vi "ClientGUIGraph.vi"() -> ()   [LabVIEW 2021]
doc: "Le protocole UDP diffère du protocole TCP car il n'y a pas de détection d'erreur avec les paquets d'informations qui sont envoyés ; il n'y a donc aucune garantie qu'un destinataire reçoive bien des données.\n\nLe protocole UDP offre la possibilité de diffuser des données sur un réseau. Spécifiez simplement une adresse IP de uns (255.255.255.255) pour essayer de diffuser l'information sur tout le réseau. Gardez à l'esprit que des routeurs et d'autres périphériques de réseau refusent généralement de diffuser au-delà de certains points, la diffusion est donc limitée dans la pratique."
panel:
  in  "Période\n(en ms)":u32(slide)=100 min=5 max=100 step=5 scale=5.0..100.0
  in  "Instruction\n[1] Get Analog\n[2] Set Digital (PWM)":u8=1 min=1 max=2
  in  "Value [0 - 255]":u8=1
  in  "Pin [0 - 11]":u8=1 max=11
  out "Request Command":u8[](array[numeric])
  out "Value":u16
  out "?":u16(graph)
  out "Response Command":u8[](array[numeric])
  in  "?":bool
  # "Version"
  # "Version"
  # "Instruction"
  # "Argument[0]"
  # "Argument[1]"
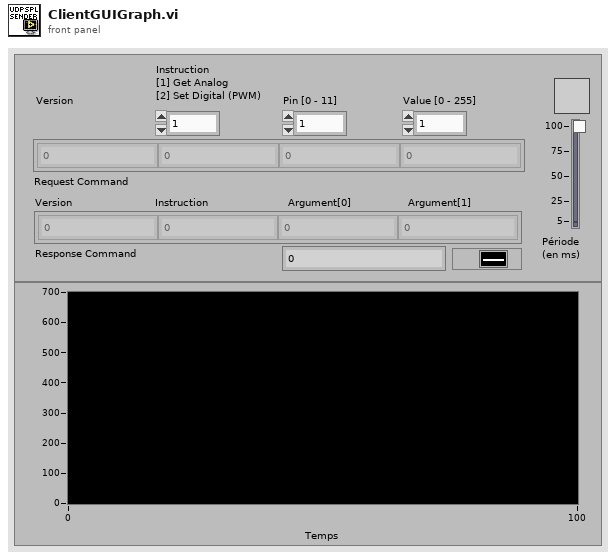
[diagram p1: front panel]
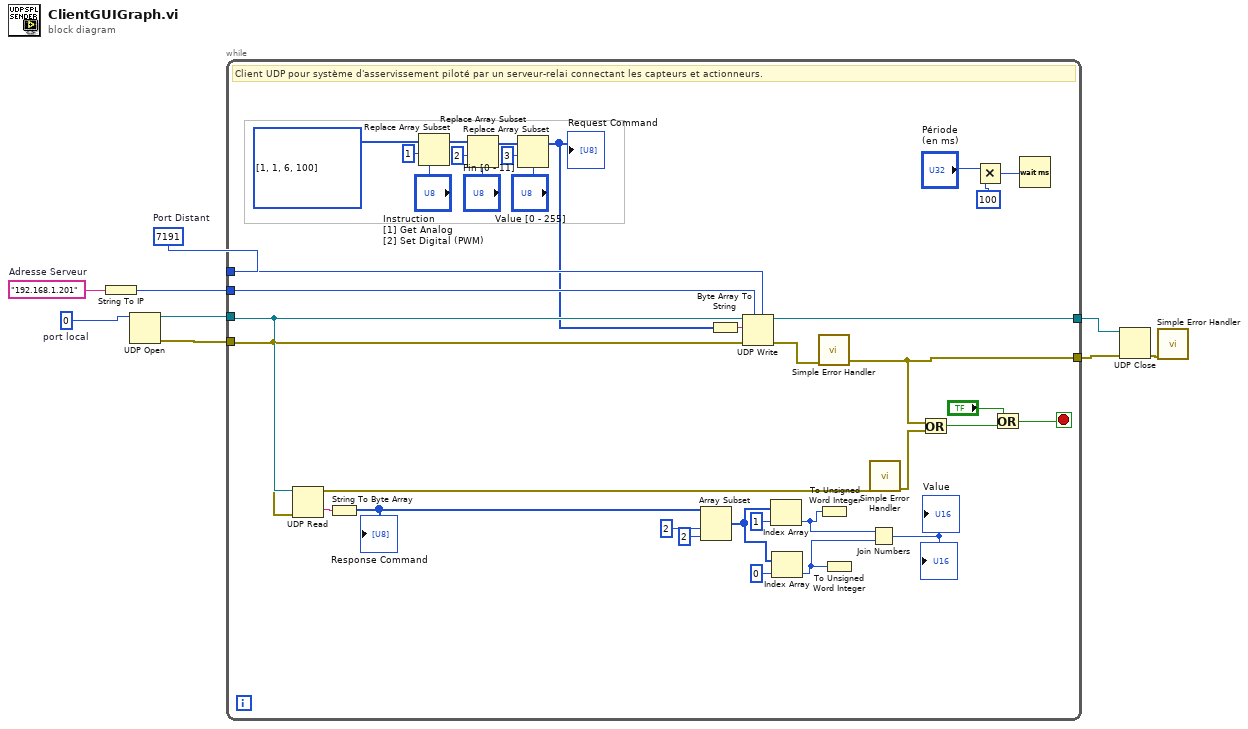
[diagram p0: block diagram]
diagram:
  w2 = u16 7191  # Port Distant
  w6 = u16 0  # port local
  w9 = "192.168.1.201"  # Adresse Serveur
  n1 = String To IP(1:w9) -> (0:w1:u32)
  n2 = UDP Open(11:w6) -> (port=w8:refnum<k16>, 0:w7:errorcluster)  [unwired: 4 in, 1 out]
  n3 = while {
    tunnel: w8 -> [w43]
    tunnel: w7 -> [w34]
    tunnel: w2 -> [w45]
    tunnel: [w29] -> w5
    tunnel: [w28] -> w4
    tunnel: w1 -> [w26]
    stop <- w27 stop-if-true
    # "Client UDP pour système d'asservissement piloté par un serveur-relai connectant les capteurs et actionneurs."
    n4 = UDP Read(connection ID=w43, 8:w34) -> (data out=w42:string, error out=w25:errorcluster)  [unwired: 2 in, 3 out]
    n5 = String To Byte Array(string=w42) -> (unsigned byte array=w10:u8[])
    "Response Command" <- w10
    n6 = Replace Array Subset(array=u8[] [1, 1, 6, 100], new element="Instruction\n[1] Get Analog\n[2] Set Digital (PWM)", index=1 ("indice")) -> (w20:u8[])
    n7 = Replace Array Subset(array=w20, new element="Pin [0 - 11]", index=2 ("indice")) -> (w19:u8[])
    n8 = Replace Array Subset(array=w19, new element="Value [0 - 255]", index=3 ("indice")) -> (w15:u8[])
    "Request Command" <- w15
    n9 = Array Subset(array=w10, index=2 ("indice"), length=2 ("longueur")) -> (w37:u8[])
    n10 = Byte Array To String(unsigned byte array=w15) -> (string=w44:string)
    n11 = UDP Write(address=w26, port or service name=w45, connection ID=w43, data in=w44, 8:w34) -> (error out=w31:errorcluster, 3:w28:refnum<k16>)  [unwired: 1 in]
    n12 = Index Array(array=w37, index=1 ("indice")) -> (element=w36:u8)
    n13 = Index Array(array=w37, index=0 ("indice")) -> (element=w35:u8)
    n14 = call <vilib>:"Simple Error Handler.vi"(9:w31) -> (6:w29:errorcluster)  [unwired: 4 in, 4 out]
    n15 = To Unsigned Word Integer(number=w36) -> ()  [unwired: 1 out]
    n16 = To Unsigned Word Integer(number=w35) -> ()  [unwired: 1 out]
    n17 = Join Numbers(hi=w36, lo=w35) -> ((hi.lo)=→"?" →"Value":u16)
    n18 = call <vilib>:"Simple Error Handler.vi"(9:w25) -> (6:w24:errorcluster)  [unwired: 4 in, 4 out]
    n19 = Or(x=w29, y=w24) -> (x .or. y?=w33:bool)
    n20 = Multiply(x="Période\n(en ms)", y=u32 100) -> (x*y=w14:u32)
    n21 = Or(x="?", y=w33) -> (x .or. y?=w27:bool)
    n22 = Wait (ms)(milliseconds to wait=w14) -> ()  [unwired: 1 out]
  }
  n23 = UDP Close(connection ID=w4, 8:w5) -> (error out=w3:errorcluster)  [unwired: 1 out]
  n24 = call <vilib>:"Simple Error Handler.vi"(9:w3) -> ()  [unwired: 4 in, 5 out]
